vi "Configure Duty Cycle.vi"(8 "error in (no error)":errorcluster, 10 "Duty Cycle (50 %)":i32=50 min=20 max=80, 11 "VISA resource name":refnum<visa-resource-name>) -> (0 "error out":errorcluster, 3 "VISA resource name out":refnum<visa-resource-name>)   [LabVIEW 2010, in "Agilent 33XXX Series.lvlib"]
doc: "Configures the duty cycle for Square waveforms."
uses:
  <instrlib>/Agilent 33XXX Series/Agilent 33XXX Series.lvlib
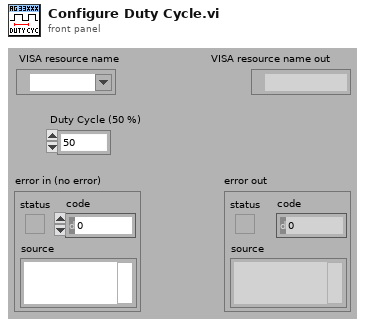
[diagram p1: front panel]
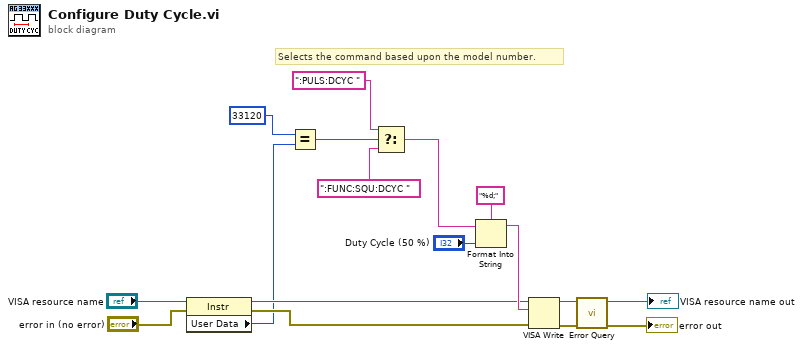
[diagram p0: block diagram]
diagram:
  # "Selects the command based upon the model number."
  n1 = property class="Instr"(reference="VISA resource name", error in="error in (no error)") -> (reference out=w11:refnum<visa-resource-name>, error out=w12:errorcluster, "User Data"=w6:u32)
  n2 = Equal?(x=u32 33120, y=w6) -> (x = y?=w8:bool)
  n3 = Select(t=":PULS:DCYC ", s=w8, f=":FUNC:SQU:DCYC ") -> (s? t:f=w9:string)
  n4 = Format Into String(format string="%d;", initial string=w9, "Duty Cycle (50 %)") -> (resulting string=w15:string)  [unwired: 1 in, 1 out]
  n5 = VISA Write(VISA resource name=w11, write buffer=w15, error in (no error)=w12) -> (VISA resource name out=w14:refnum<visa-resource-name>, error out=w13:errorcluster)  [unwired: 1 out]
  n6 = call <instrlib>:"Error Query.vi"("error in (no error)"=w13, "VISA resource name"=w14) -> ("error out"=→"error out":errorcluster, "VISA resource name out"=→"VISA resource name out":refnum<visa-resource-name>)  [unwired: 6 in, 2 out]
